vi "Process IMAQ Image.vi"() -> ()   [LabVIEW 2020]
uses:
  6d5f1638-640c-4e20-b011-0cee3ae60b95.vi
  688a6956-cd2d-4b8a-a8be-e172edc5432f.vi
  45820c2d-b3f1-45d5-9983-17417cdda85c.vi
  G-Embedded-Python-Interpreter-Toolkit/Null Py Object Refnum.vi
  6d5f1638-640c-4e20-b011-0cee3ae60b95.vi/96ddca92-7bbf-40e2-a1a5-d32f291eb6af.vi
  G-Embedded-Python-Interpreter-Toolkit-IMAQ/IMAQ to Py Object.vi/22f05568-5bba-4402-9e98-aca160827363.vi
  688a6956-cd2d-4b8a-a8be-e172edc5432f.vi/6c7a13f1-33d3-431d-8188-904cac5422b3.vi
  45820c2d-b3f1-45d5-9983-17417cdda85c.vi/6c7a13f1-33d3-431d-8188-904cac5422b3.vi
  G-Embedded-Python-Interpreter-Toolkit/Python Object Reference to Pointer Sized Ref.vi
  G-Embedded-Python-Interpreter-Toolkit/Pointer Sized Ref to Python Object Reference.vi
  G-Embedded-Python-Interpreter-Toolkit/Merge Call Library Errors.vi
  G-Embedded-Python-Interpreter-Toolkit/Generate Argument Type Info.vi
  G-Embedded-Python-Interpreter-Toolkit/Create Py Object IMAQ Image.vi
  G-Embedded-Python-Interpreter-Toolkit/G-Embedded-Python-Interpreter-Toolkit.lvlib
  G-Embedded-Python-Interpreter-Toolkit-IMAQ/G-Embedded-Python-Interpreter-Toolkit-IMAQ.lvlib
panel:
  out "Image":T1(plugin-control)
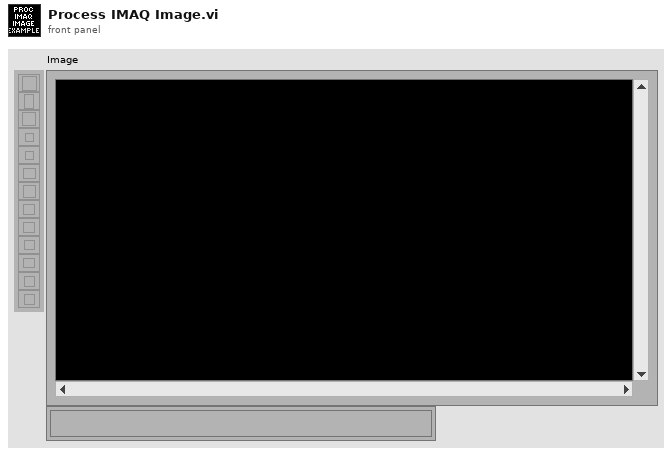
[diagram p1: front panel]
types:
  T1 = typedef "IMAQ Image.ctl" = refnum<image>
  T2 = typedef "Image Type" = u32
  T3 = typedef "G-Embedded-Python-Interpreter-Toolkit.lvlib/Python Object Reference.ctl" = refnum<k1>
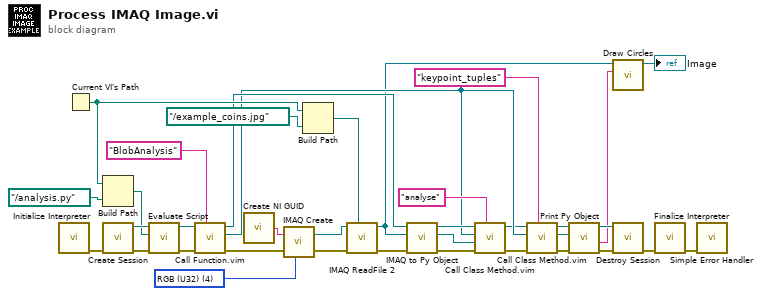
[diagram p0: block diagram]
diagram:
  w23 = T2 4 items=["Grayscale (U8)", "Grayscale (I16)", "Grayscale (SGL)", "Complex (CSG)", "RGB (U32)", "HSL (U32)", "RGB (U64)", "Grayscale (U16)"] ("Image Type")
  n1 = call "Initialize Interpreter.vi"() -> ("error out"=w36:errorcluster)  [unwired: 10 in, 1 out]
  n2 = Current VI's Path() -> (path=w21:path)
  n3 = Build Path(base path=w21, name or relative path=path "../analysis.py") -> (appended path=w32:path)
  n4 = call "Create Session.vi"("error in (no error)"=w36) -> ("error out"=w35:errorcluster, "Session Handle"=w34:refnum<data-value>)  [unwired: 9 in]
  n5 = call "Evaluate Script.vi"("error in (no error)"=w35, "Script File Path"=w32, "Session Handle in"=w34) -> ("error out"=w29:errorcluster, "Session Handle out"=w30:refnum<data-value>)  [unwired: 7 in]
  n6 = call "Call Function.vim"("Function Name"="BlobAnalysis", "error in (no error)"=w29, "Data Value Reference in"=w30) -> ("error out"=w22:errorcluster, "Returned Python Object Refnum"=w11:T3, "Data Value Reference out"=w18:refnum<data-value>)  [unwired: 6 in]
  n7 = call <vilib>:"Create NI GUID.vi"() -> ("NI GUID"=w13:string)
  n8 = call "IMAQ Create"("Image Name"=w13, "Image Type"=w23, "error in (no error)"=w22) -> ("New Image"=w24:T1, "error out"=w25:errorcluster)  [unwired: 2 in]
  n9 = Build Path(base path=w21, name or relative path=path "../example_coins.jpg") -> (appended path=w19:path)
  n10 = call "IMAQ ReadFile 2"("File Path"=w19, "error in (no error)"=w25, "Image"=w24) -> ("error out"=w17:errorcluster, "Image Out"=w2:T1)  [unwired: 4 in, 3 out]
  n11 = call "IMAQ to Py Object.vi"("error in (no error)"=w17, "Image In"=w2, "Session Handle in"=w18) -> ("error out"=w15:errorcluster, "Python Object Refnum"=w14:T3, "Session Handle out"=w16:refnum<data-value>)  [unwired: 6 in]
  n12 = call "Call Class Method.vim"("Function Name"="analyse", "error in (no error)"=w15, "Arguments in (Default - Empty)"=w14, "Class Instance"=w11, "Data Value Reference in"=w16) -> ("error out"=w12:errorcluster, "Data Value Reference out"=w7:refnum<data-value>)  [unwired: 4 in, 1 out]
  n13 = call "Call Class Method.vim"("Function Name"="keypoint_tuples", "error in (no error)"=w12, "Class Instance"=w11, "Data Value Reference in"=w7) -> ("error out"=w10:errorcluster, "Returned Python Object Refnum"=w8:T3, "Data Value Reference out"=w6:refnum<data-value>)  [unwired: 5 in]
  n14 = call "Print Py Object.vi"("error in (no error)"=w10, "Python Object Refnum in"=w8, "Session Handle in"=w6) -> ("error out"=w4:errorcluster, "Print Ouptut"=w3:string, "Session Handle out"=w5:refnum<data-value>)  [unwired: 5 in, 1 out]
  n15 = call "Draw Circles.vi"("Print Ouptut"=w3, "Refnum in"=w2) -> ("Refnum out"=→"Image":T1)  [unwired: 9 in]
  n16 = call "Destroy Session.vi"("error in (no error)"=w4, "Session Handle"=w5) -> ("error out"=w28:errorcluster)  [unwired: 9 in]
  n17 = call "Finalize Interpreter.vi"("error in (no error)"=w28) -> ("error out"=w27:errorcluster)  [unwired: 10 in]
  n18 = call <vilib>:"Simple Error Handler.vi"("error in (no error)"=w27) -> ()  [unwired: 4 in, 5 out]
